vi "Intake Maniford Dynamics.vi"(9 "dt":sgl=1.0 format="%0.2f", 10 "Engine Speed (rad/s)":sgl, 11 "Air Mass Flow from Throttle (g/s)":sgl) -> (1 "Air Mass/Cycle (g)":sgl, 2 "Manifold Pressure (bar)":sgl format="%0.2f", 3 "Air Mass Flow to Cylinder (g/s)":sgl)   [LabVIEW 2016, in "NI-PCG Vehicle Model.lvlib"]
uses:
  NI-PCG Vehicle Model.lvlib
  Globals/Parameters.vi
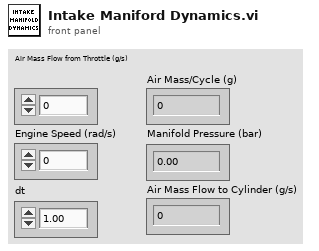
[diagram p1: front panel]
types:
  T1 = typedef "NI-PCG Vehicle Model.lvlib/Engine Parameters.ctl" = cluster{"Ambient Parameters":cluster{"Temperature (K)":sgl, "Pressure (Pa)":sgl}, "Air Parameters":cluster{"R (Ideal Gas Constant)":sgl, "Molecular Weight":sgl, "Cp (Specific Heat Constant)":sgl, "Density (kg/m^3)":sgl, "Stoichiometric A/F Ratio":sgl}, "Engine Geometry Parameters":cluster{"Cylinder Volume (l)":sgl, "J (Rotational Moment of Inertia)":sgl, "Minimuim Engine Speed":sgl, "Maximum Engine Speed":sgl, "Intake Manifold Volume (l)":sgl}, "Volumetric Efficiency Map":cluster{"MAP":sgl[], "RPM":sgl[], "Table":sgl[][]}, "Fuel LHV (J/kg)":sgl, "Combustion Efficiency Map":cluster{"Spark Timing (deg BTDC))":sgl[], "Engine Speed (RPM)":sgl[], "Combustion Efficiency":sgl[][]}, "Thermodynamic Efficiency":sgl}
  T2 = typedef "NI-PCG Vehicle Model.lvlib/Transmission Parameters.ctl" = cluster{"Final Drive Ratio":sgl, "Transmission Gear Ratios":cluster{"Gears":sgl[], "Gear Ratios":sgl[]}, "Torque Converter Map":cluster{"Speed Ratio":sgl[], "K Factor":sgl[], "Torque Ratio":sgl[]}, "Upshift Throttle":sgl[], "Downshift Throttle":sgl[], "Upshift Table":sgl[][], "Downshift Table":sgl[][], "Wait Time":u8}
  T3 = typedef "NI-PCG Vehicle Model.lvlib/Vehicle Parameters.ctl" = cluster{"Vehicle Mass (kg)":sgl, "Vehicle Cd":sgl, "Vehicle Frontal Area (m^2)":sgl, "Wheel Radius (m)":sgl, "Wheel Rolling Resistance":sgl}
  T4 = cluster{"Engine Parameters":T1, "Transmission Parameters":T2, "Vehicle Parameters":T3}
  T5 = cluster{"MAP":sgl[], "RPM":sgl[], "Table":sgl[][]}
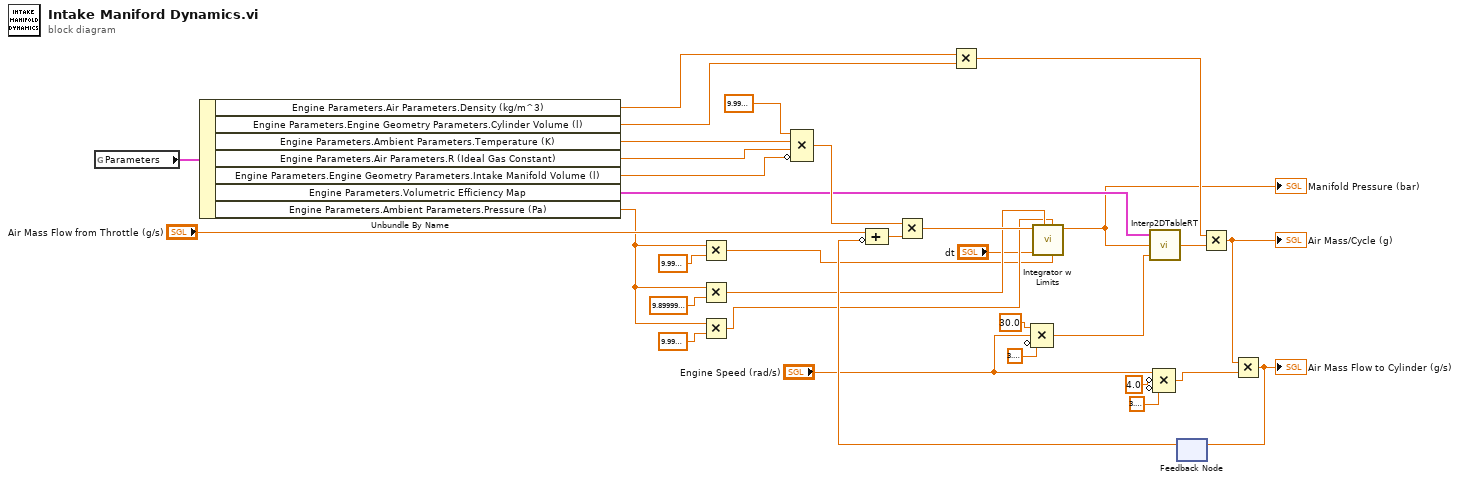
[diagram p0: block diagram]
diagram:
  n1 = global read "Parameters.vi" "Parameters"() -> (w10:T4)
  n2 = Unbundle By Name(w10) -> ("Engine Parameters.Air Parameters.Density (kg/m^3)"=w7:sgl, "Engine Parameters.Engine Geometry Parameters.Cylinder Volume (l)"=w8:sgl, "Engine Parameters.Ambient Parameters.Temperature (K)"=w21:sgl, "Engine Parameters.Air Parameters.R (Ideal Gas Constant)"=w19:sgl, "Engine Parameters.Engine Geometry Parameters.Intake Manifold Volume (l)"=w20:sgl, "Engine Parameters.Volumetric Efficiency Map"=w18:T5, "Engine Parameters.Ambient Parameters.Pressure (Pa)"=w9:sgl)
  n3 = Multiply(x=w9, y=sgl 1e-06) -> (x*y=w3:sgl)
  n4 = Multiply(x=w9, y=sgl 9.9e-06) -> (x*y=w5:sgl)
  n5 = Multiply(x=w9, y=sgl 1e-08) -> (x*y=w4:sgl)
  n6 = Compound Arithmetic op=MULTIPLY(sgl 1e-05 ("value"), w21, w19, invert w20) -> (w28:sgl)
  n7 = Multiply(x=w7, y=w8) -> (x*y=w26:sgl)
  n8 = Compound Arithmetic op=MULTIPLY(sgl 30.0 ("value"), "Engine Speed (rad/s)", invert sgl 3.1415927) -> (w12:sgl)
  n9 = Compound Arithmetic op=MULTIPLY("Engine Speed (rad/s)", invert sgl 4.0 ("value"), invert sgl 3.1415927) -> (w24:sgl)
  n10 = feedback #1() -> (w22:sgl)  [unwired: 1 in]
  n11 = Compound Arithmetic op=ADD("Air Mass Flow from Throttle (g/s)", invert w22) -> (w32:sgl)
  n12 = Multiply(x=w28, y=w32) -> (x*y=w6:sgl)
  n13 = call "Integrator w Limits.vi"("Initial Condition"=w3, "lower limit"=w4, "upper limit"=w5, "dt [s]"="dt", "x"=w6) -> ("Result"=w1:sgl)  [unwired: 6 in]
  "Manifold Pressure (bar)" <- w1
  n14 = call <vilib>:"Interp2DTableRT.vi"("Y"=w12, "X"=w1, "2DTable"=w18) -> ("Z"=w11:sgl)
  n15 = Multiply(x=w26, y=w11) -> (x*y=w25:sgl)
  "Air Mass/Cycle (g)" <- w25
  n16 = Multiply(x=w25, y=w24) -> (x*y=w23:sgl)
  "Air Mass Flow to Cylinder (g/s)" <- w23
  n17 = feedback-in #1(w23) -> ()
